vi "scale to u8 no histogram.vi"(11 "Input":sgl[](array[numeric])) -> (3 "Output":sgl[](array[numeric]))   [LabVIEW 2013]
panel:
  out "10% min value":sgl
  out "old min value":sgl
  out "old max value":sgl
  out "10% max value":sgl
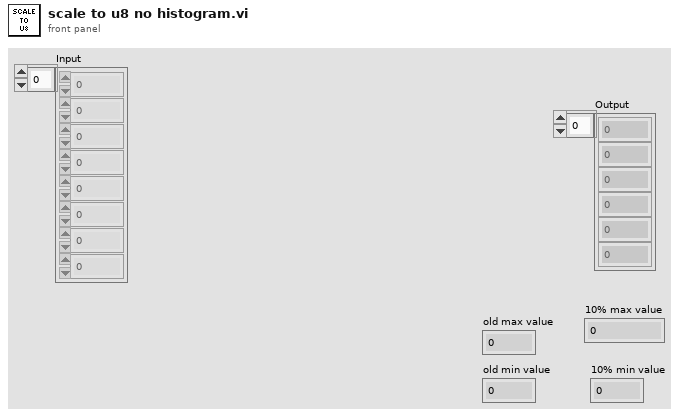
[diagram p1: front panel]
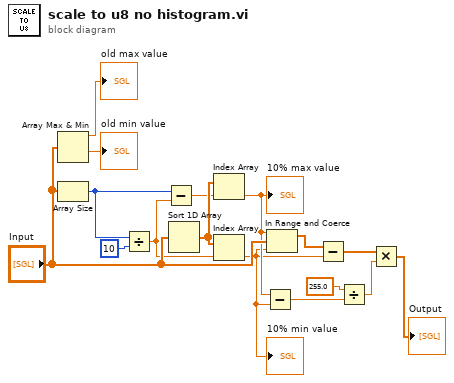
[diagram p0: block diagram]
diagram:
  n1 = Array Max & Min(array="Input") -> (max value=→"old max value":sgl, min value=→"old min value":sgl)  [unwired: 2 out]
  n2 = Array Size(array="Input") -> (size(s)=w5:i32)
  n3 = Divide(x=w5, y=10) -> (x/y=w4:dbl)
  n4 = Subtract(x=w5, y=w4) -> (x-y=w3:dbl)
  n5 = Sort 1D Array(array="Input") -> (sorted array=w6:sgl[])
  n6 = Index Array(array=w6, index=w3) -> (element=w2:sgl)
  "10% max value" <- w2
  n7 = Index Array(array=w6, index=w4) -> (element=w1:sgl)
  "10% min value" <- w1
  n8 = Subtract(x=w2, y=w1) -> (x-y=w12:sgl)
  n9 = In Range and Coerce(upper limit=w2, x="Input", lower limit=w1) -> (coerced(x)=w13:sgl[])  [unwired: 1 out]
  n10 = Subtract(x=w13, y=w1) -> (x-y=w10:sgl[])
  n11 = Divide(x=sgl 255.0, y=w12) -> (x/y=w9:sgl)
  n12 = Multiply(x=w10, y=w9) -> (x*y=→"Output":sgl[])
